vi "Validate Path.vi"(0 "input path":path, 11 "error in":errorcluster) -> (4 "validated path":path, 8 "warning":string, 15 "error out":errorcluster)   [LabVIEW 2021, in "Converter.lvlib"]
uses:
  Converter.lvlib
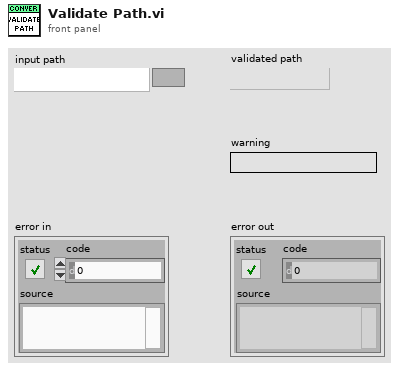
[diagram p1: front panel]
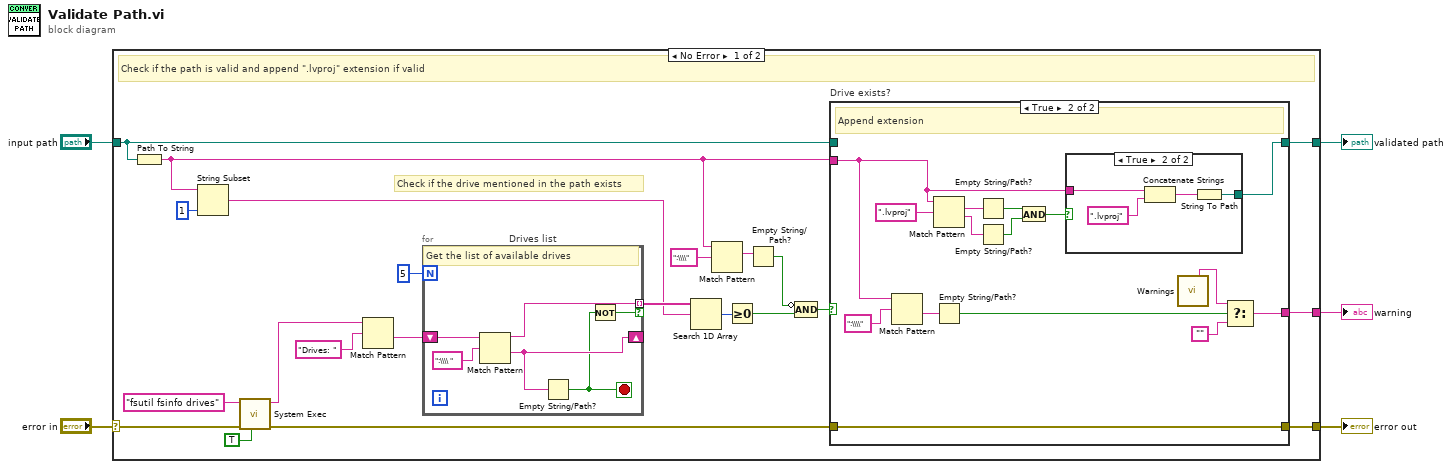
[diagram p0: block diagram]
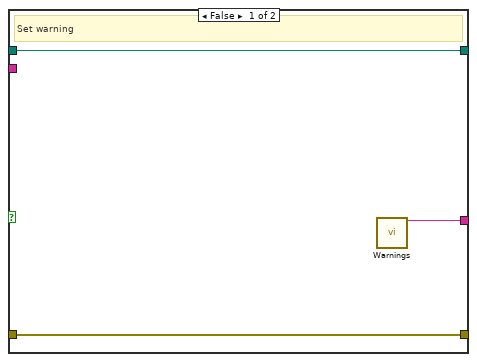
[diagram p2: hidden frame]
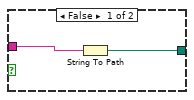
[diagram p3: hidden frame]
diagram:
  n1 = case shown="No Error" "error in" {
    selector: "error in" -> [w27 w59]
    tunnel: "input path" -> [w15 w58]
    tunnel: [w17 w59] -> w3
    tunnel: [w16 _] -> w2
    tunnel: [w14 w58] -> w1
    frame No Error {
      # "Check if the drive mentioned in the path exists"
      # "Check if the path is valid and append \".lvproj\" extension if valid"
      n2 = Path To String(path=w15) -> (string=w10:string)
      n3 = String Subset(string=w10, length (rest)=1 ("length (rest)")) -> (substring=w19:string)  [unwired: 1 in]
      n4 = call <vilib>:"System Exec.vi"("run minimized? (F)"=TRUE, "error in (no error)"=w27, "command line"="fsutil fsinfo drives") -> ("error out"=w13:errorcluster, "standard output"=w24:string)  [unwired: 5 in, 2 out]
      n5 = Match Pattern(string=w24, regular expression="Drives: ") -> (after substring=w22:string)  [unwired: 1 in, 3 out]
      n6 = for "Drives list" {
        N: 5 -> [_]
        tunnel: [w31] -> w20 mode=indexing if=w28
        shift-right: [w30] -> _
        shift-left: w22 -> [w33]
        stop <- w29 stop-if-true
        # "Get the list of available drives"
        n7 = Match Pattern(string=w33, regular expression=":\\\\ ") -> (before substring=w31:string, after substring=w30:string)  [unwired: 1 in, 2 out]
        n8 = Empty String/Path?(string/path=w30) -> (empty?=w29:bool)
        n9 = Not(x=w29) -> (.not. x?=w28:bool)
      }
      n10 = Search 1D Array(1D array=w20, element=w19) -> (index of element=w18:i32)  [unwired: 1 in]
      n11 = Match Pattern(string=w10, regular expression=":\\\\") -> (match substring=w9:string)  [unwired: 1 in, 3 out]
      n12 = Greater Or Equal To 0?(x=w18) -> (x >= 0?=w8:bool)
      n13 = Empty String/Path?(string/path=w9) -> (empty?=w7:bool)
      n14 = Compound Arithmetic op=AND(invert w7, w8) -> (w6:bool)
      n15 = case "Drive exists?" shown="True" w6 {
        tunnel: [w35 w51] -> w17
        tunnel: w13 -> [w35 w51]
        tunnel: [w36 w46] -> w16
        tunnel: [w34 w50] -> w14
        tunnel: w15 -> [w34 _]
        tunnel: w10 -> [_ w43]
        frame False {
          # "Set warning"
          n16 = call "Warnings.vi"() -> ("invalid project path"=w36:string)  [unwired: 8 in, 7 out]
        }
        frame True {
          # "Append extension"
          n17 = Match Pattern(string=w43, regular expression=":\\\\") -> (after substring=w48:string)  [unwired: 1 in, 3 out]
          n18 = Match Pattern(string=w43, regular expression=".lvproj") -> (match substring=w41:string, after substring=w40:string)  [unwired: 1 in, 2 out]
          n19 = Empty String/Path?(string/path=w48) -> (empty?=w44:bool)
          n20 = Empty String/Path?(string/path=w41) -> (empty?=w39:bool)
          n21 = Empty String/Path?(string/path=w40) -> (empty?=w38:bool)
          n22 = And(x=w39, y=w38) -> (x .and. y?=w37:bool)
          n23 = case shown="True" w37 {
            tunnel: [w52 w55] -> w50
            tunnel: w43 -> [w53 w54]
            frame False {
              n24 = String To Path(string=w53) -> (path=w52:path)
            }
            frame True {
              n25 = Concatenate Strings(w54, ".lvproj" ("string")) -> (w56:string)
              n26 = String To Path(string=w56) -> (path=w55:path)
            }
          }
          n27 = call "Warnings.vi"() -> ("project name"=w45:string)  [unwired: 8 in, 7 out]
          n28 = Select(t=w45, s=w44, f="") -> (s? t:f=w46:string)
        }
      }
    }
    frame Error {
      # "Pass"
    }
  }
  "error out" <- w3
  "warning" <- w2
  "validated path" <- w1
